vi "Read BMS LV Status Loop.vi"(7 "timeout in ms (-1)":i32=-1, 8 "error in":errorcluster, 9 "Error Queue":refnum<queue>, 11 "CAN Session In":T2=refnum) -> (2 "BMS Low Voltage Status":T1 {"Temp. 0" scale=0.0..100.0; "Temp. 1" scale=0.0..100.0}, 3 "CAN Session Out":T2)   [LabVIEW 2016]
uses:
  Program Files (x86)/National Instruments/LabVIEW 2016/examples/robotics/EPOS2 CANOpen Driver/Low Level VIs/Typedefs/CAN Refnum.ctl
  Program Files (x86)/National Instruments/LabVIEW 2016/examples/robotics/EPOS2 CANOpen Driver/Low Level VIs/Typedefs/CAN Session Pointer.ctl
  Program Files (x86)/National Instruments/LabVIEW 2016/examples/robotics/EPOS2 CANOpen Driver/Low Level VIs/Typedefs/CAN Communication References.ctl
  Program Files (x86)/National Instruments/LabVIEW 2016/examples/robotics/EPOS2 CANOpen Driver/Low Level VIs/Typedefs/kill process notifier array.ctl
  Program Files (x86)/National Instruments/LabVIEW 2016/examples/robotics/EPOS2 CANOpen Driver/Low Level VIs/Typedefs/Write Queue.ctl
  Program Files (x86)/National Instruments/LabVIEW 2016/examples/robotics/EPOS2 CANOpen Driver/Low Level VIs/Typedefs/FPGA CAN Frame Cluster.ctl
  RT/BMS Voltage status 2.ctl
  RT/Read single CAN.vi
  RT/Data to LV BMS Status.vi
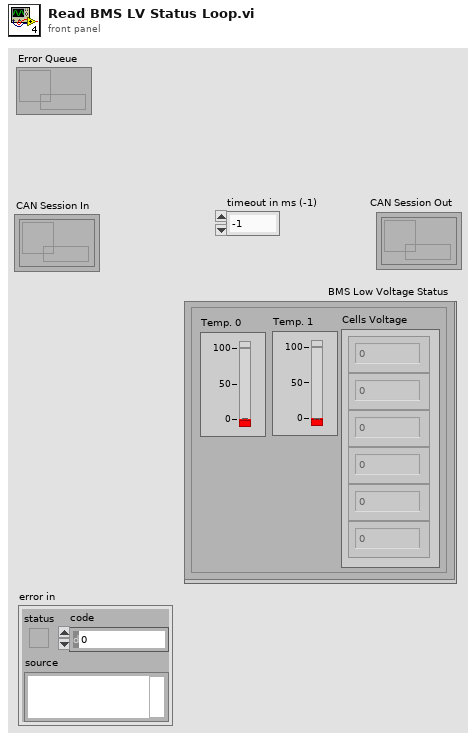
[diagram p1: front panel]
types:
  T1 = typedef "BMS Voltage status 2.ctl" = cluster{"Cells Voltage":dbl[], "Temp. 1":u8, "Temp. 0":u8}
  T2 = typedef "CAN Refnum.ctl" = refnum<k1>
  T3 = typedef "FPGA CAN Frame Cluster.ctl" = cluster{"Timestamp":u64, "Identifier":u32, "Type":u8, "InfoA":u8, "InfoB":u8, "DataLength":u8, "Data":u8[]}
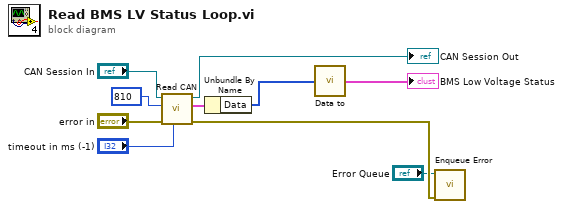
[diagram p0: block diagram]
diagram:
  n1 = call-poly "Read CAN.vi"("timeout in ms (-1)"="timeout in ms (-1)", "error in"="error in", "ID"=810 ("Data 0"), "CAN Session In"="CAN Session In") -> ("error out"=w2:errorcluster, "CAN Frame Out"=w10:T3, "CAN Session Out"=→"CAN Session Out":T2)  [unwired: 5 in]
  n2 = Unbundle By Name(w10) -> ("Data"=w9:u8[])
  n3 = call-poly "Data to.vi"("Data"=w9) -> ("BMS Low Voltage Status"=→"BMS Low Voltage Status":T1)
  n4 = call "Enqueue Error.vi"("error in"=w2, "Error Queue"="Error Queue") -> ()  [unwired: 10 in]
